vi "RESTful INI Build RegEx String.vi"() -> (0 "keyword format (RegEx)":string)   [LabVIEW 2020]
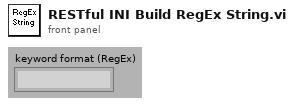
[diagram p1: front panel]
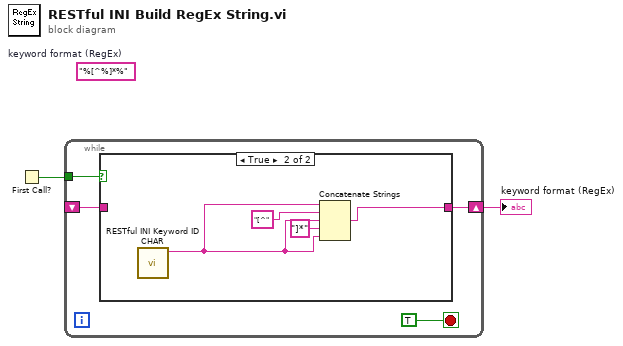
[diagram p0: block diagram]
diagram:
  (unwired) "%[^%]*%"  # keyword format (RegEx)
  n1 = First Call?() -> (First Call?: T/F=w2:bool)
  n2 = while {
    tunnel: w2 -> [w6]
    shift-right: [w3] -> w1
    shift-left: _ -> [w5]
    stop <- TRUE stop-if-true
    n3 = case shown="True" w6 {
      tunnel: w5 -> [w7 _]
      tunnel: [w7 w8] -> w3
      frame False {
      }
      frame True {
        n4 = call <vilib>:"RESTful INI Keyword ID CHAR.vi"() -> ("Keyword ID CHAR"=w9:string)  [unwired: 11 in]
        n5 = Concatenate Strings(w9, "[^" ("string"), w9, "]*" ("string"), w9) -> (w8:string)
      }
    }
  }
  "keyword format (RegEx)" <- w1
